vi "Byte Array Checksum.vi"(1 "Number of Values":i32, 3 "Byte Array":u8[](array[numeric]) format="%02x") -> (0 "Checksum":u8 format="%02x")   [LabVIEW 2010]
doc: "Returns the sum of the first <b>Number of Values</b> in a byte array."
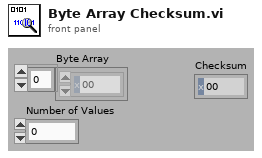
[diagram p1: front panel]
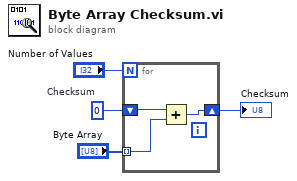
[diagram p0: block diagram]
diagram:
  w3 = u8 0  # Checksum
  n1 = for {
    N: "Number of Values" -> [_]
    tunnel: "Byte Array" -> [w6] mode=indexing
    shift-right: [w5] -> w1
    shift-left: w3 -> [w7]
    n2 = Add(x=w7, y=w6) -> (x+y=w5:u8)
  }
  "Checksum" <- w1
